vi "PI Control Anti Windup.vi"(3 "bsp":dbl, 4 "ki":dbl, 5 "kp":dbl, 6 "y":dbl, 7 "r":dbl) -> (1 "u":dbl)   [LabVIEW 2018]
doc: "Proportional-integral (PI) controller."
uses:
  <vilib>/Simulation/Implementation/Shared/SIMSCR Execution Mode.ctl
  <vilib>/Simulation/Scripting/Companion Diagram/SimConfigNode/SimParams.ctl
  <vilib>/Simulation/Scripting/Companion Diagram/SimConfigNode/_simSolvers.ctl
  <vilib>/Simulation/Param Hierarchy/Typedefs/SIMPH Param Control Actions.ctl
  <vilib>/Simulation/Implementation/Shared/SIM limit type.ctl
  <vilib>/Simulation/Implementation/Shared/NILVSim_ParamChanged.vi
  <vilib>/Simulation/Implementation/Shared/NILVSIM_BeginStep.vi
  <vilib>/Simulation/SignalArithmetic/Implementation/NILVSim Gain.llb/SIM Gain (scalar).vi
  <vilib>/Simulation/ContinuousLinear/Implementation/NILVSim Integrator new.llb/SIM Integrator distributor (scalar).vi
  <vilib>/Simulation/ContinuousLinear/Implementation/NILVSim Integrator new.llb/SIM Integrator collector (scalar).vi
  <vilib>/Simulation/Implementation/Shared/NILVSim_Manager.vi
  <vilib>/Utility/error.llb/Clear Errors.vi
  <vilib>/Simulation/Implementation/Shared/NILVSim_FinalizeModel.vi
  <vilib>/Simulation/Implementation/Shared/SIM Unbundle Sim Info.vi
  <vilib>/Simulation/Implementation/Shared/SIMSH Read Queue.vi
  <vilib>/Simulation/Implementation/Shared/NILVSim_Initialize.vi
  <vilib>/Simulation/Utility/Implementation/NILVSim Get Time and IsAcceptedStep.vi
  <vilib>/Simulation/Implementation/Shared/NILVSim_GetModelError.vi
  <vilib>/Simulation/Implementation/Shared/SIM SimErrorHandler.vi
  <vilib>/Simulation/Implementation/Shared/SIM Bundle Sim Info.vi
  <vilib>/Simulation/Scripting/Companion Diagram/SimConfigNode/SimDog.xnode
  <vilib>/Simulation/Implementation/XNodeFramework/SimXNode/SimX.xnode
  <vilib>/Simulation/ContinuousLinear/Implementation/NILVSim Integrator new.llb/SIM Integrator (scalar).vi
  <vilib>/Simulation/Implementation/Shared/NI_SIM_Implementation.lvlib
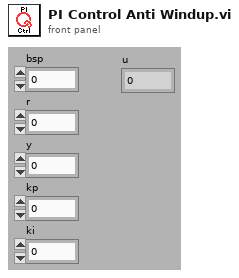
[diagram p1: front panel]
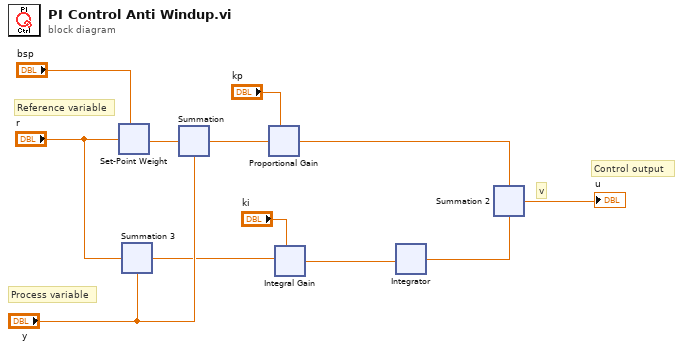
[diagram p0: block diagram]
diagram:
  # "v"
  # "Control output"
  # "Process variable"
  # "Reference variable"
  n1 = xnode "Set-Point Weight"("gain"="bsp", "input"="r") -> ("output"=w4:dbl)  [unwired: 2 in]
  n2 = xnode ("Summation 3")("Operand1"="r", "Operand2"="y") -> ("Result"=w6:dbl)
  n3 = xnode ("Summation")("Operand1"=w4, "Operand2"="y") -> ("Result"=w9:dbl)
  n4 = xnode "Proportional Gain"("gain"="kp", "input"=w9) -> ("output"=w10:dbl)  [unwired: 2 in]
  n5 = xnode "Integral Gain"("gain"="ki", "input"=w6) -> ("output"=w2:dbl)  [unwired: 2 in]
  n6 = xnode ("Integrator")("input"=w2) -> ("output"=w7:dbl)  [unwired: 9 in, 2 out]
  n7 = xnode ("Summation 2")("Operand1"=w10, "Operand2"=w7) -> ("Result"=→"u":dbl)
